vi "default_JSON.vi"(8 "error in (no error)":errorcluster, 11 "SecureMqttCodec in":refnum<class "SecureMqttCodec.lvclass">) -> (0 "error out":errorcluster, 3 "SecureMqttCodec out":refnum<class "SecureMqttCodec.lvclass">)   [LabVIEW 2020, in "SecureMqttCodec.lvclass"]
uses:
  SecureMqttCodec.lvclass
  <vilib>/addons/JSON API/Get Polymorphic/JSON GetSet.lvlib
  <vilib>/addons/JSON API/JSON Value/JSON Value.lvclass
  <vilib>/addons/JSON API/JSON Scalar/Set String.vi
  <vilib>/addons/JSON API/JSON Scalar/JSON Scalar.lvclass
  <vilib>/addons/JSON API/JSON Array/Set JSON Array.vi
  <vilib>/addons/JSON API/JSON Array/JSON Array.lvclass
  <vilib>/addons/JSON API/JSON Value/Set from JSON string.vi
  <vilib>/addons/JSON API/JSON Value/Get Array by name.vi
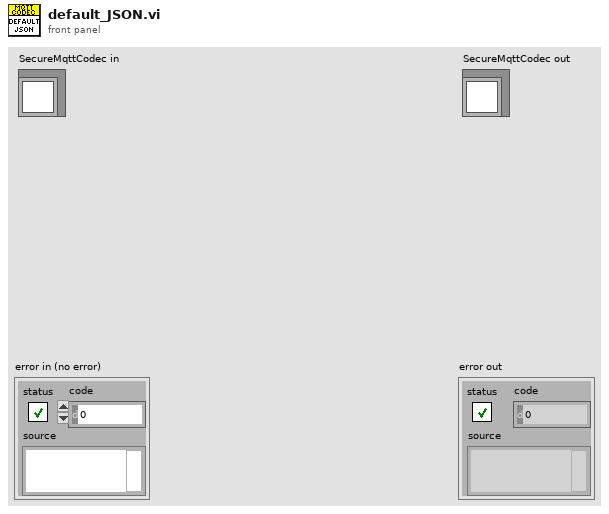
[diagram p1: front panel]
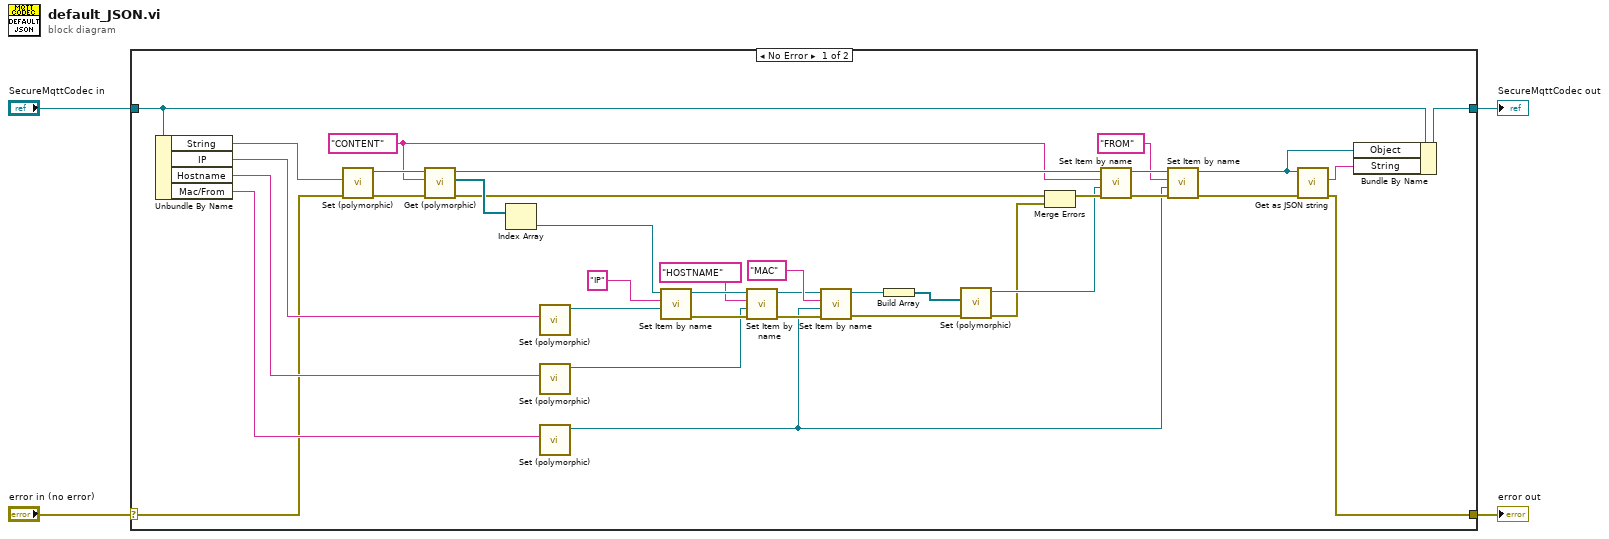
[diagram p0: block diagram]
diagram:
  n1 = case shown="No Error" "error in (no error)" {
    selector: "error in (no error)" -> [w11 w43]
    tunnel: [w10 w43] -> w3
    tunnel: [w13 w42] -> w1
    tunnel: "SecureMqttCodec in" -> [w41 w42]
    frame No Error {
      w14 = "CONTENT" ("name")
      n2 = Unbundle By Name(w41) -> ("String"=w32:string, "IP"=w31:string, "Hostname"=w30:string, "Mac/From"=w29:string)
      n3 = call-poly <vilib>:"Set (polymorphic).vi"("error in (no error)"=w11, "JSON stream"=w32) -> ("error out"=w39:errorcluster, "JSON Value out"=w36:refnum<class "JSON Value.lvclass">)  [unwired: 7 in, 1 out]
      n4 = call-poly <vilib>:"Get (polymorphic).vi"("error in (no error)"=w39, "name"=w14, "JSON Value In"=w36) -> ("error out"=w18:errorcluster, "Array"=w37:refnum<class "JSON Value.lvclass">[], "JSON Value Out"=w17:refnum<class "JSON Value.lvclass">)  [unwired: 5 in, 1 out]
      n5 = Index Array(array=w37) -> (element=w38:refnum<class "JSON Value.lvclass">)  [unwired: 1 in]
      n6 = call-poly <vilib>:"Set (polymorphic).vi"("String"=w31) -> ("JSON Scalar out"=w33:refnum<class "JSON Scalar.lvclass">)  [unwired: 9 in, 1 out]
      n7 = call-poly <vilib>:"Set (polymorphic).vi"("String"=w30) -> ("JSON Scalar out"=w35:refnum<class "JSON Scalar.lvclass">)  [unwired: 9 in, 1 out]
      n8 = call-poly <vilib>:"Set (polymorphic).vi"("String"=w29) -> ("JSON Scalar out"=w5:refnum<class "JSON Scalar.lvclass">)  [unwired: 9 in, 1 out]
      n9 = call-dynamic "Set Item by name.vi"("Value"=w33, "name"="IP", "JSON Value In"=w38) -> ("error out"=w40:errorcluster, "JSON Value Out"=w34:refnum<class "JSON Value.lvclass">)  [unwired: 6 in, 1 out]
      n10 = call-dynamic "Set Item by name.vi"("error in (no error)"=w40, "Value"=w35, "name"="HOSTNAME", "JSON Value In"=w34) -> ("error out"=w24:errorcluster, "JSON Value Out"=w25:refnum<class "JSON Value.lvclass">)  [unwired: 5 in, 1 out]
      n11 = call-dynamic "Set Item by name.vi"("error in (no error)"=w24, "Value"=w5, "name"="MAC", "JSON Value In"=w25) -> ("error out"=w21:errorcluster, "JSON Value Out"=w22:refnum<class "JSON Value.lvclass">)  [unwired: 5 in, 1 out]
      n12 = Build Array(w22) -> (w23:refnum<class "JSON Value.lvclass">[])
      n13 = call-poly <vilib>:"Set (polymorphic).vi"("error in (no error)"=w21, "Array"=w23) -> ("error out"=w15:errorcluster, "JSON Array out"=w16:refnum<class "JSON Array.lvclass">)  [unwired: 8 in]
      n14 = Merge Errors(w18, w15) -> (w20:errorcluster)
      n15 = call-dynamic "Set Item by name.vi"("error in (no error)"=w20, "Value"=w16, "name"=w14, "JSON Value In"=w17) -> ("error out"=w19:errorcluster, "JSON Value Out"=w8:refnum<class "JSON Value.lvclass">)  [unwired: 5 in, 1 out]
      n16 = call-dynamic "Set Item by name.vi"("error in (no error)"=w19, "Value"=w5, "name"="FROM", "JSON Value In"=w8) -> ("error out"=w9:errorcluster, "JSON Value Out"=w7:refnum<class "JSON Value.lvclass">)  [unwired: 5 in, 1 out]
      n17 = call <vilib>:"Get as JSON string.vi"("error in (no error)"=w9, "JSON Value in"=w7) -> ("error out"=w10:errorcluster, "<JSON>"=w12:string)  [unwired: 8 in]
      n18 = Bundle By Name(cluster=w41, "Object"=w7, "String"=w12) -> (w13:refnum<class "SecureMqttCodec.lvclass">)
    }
    frame Error {
    }
  }
  "error out" <- w3
  "SecureMqttCodec out" <- w1
